vi "Calc Currente Exposure Time.vi"(8 "error in (no error)":errorcluster, 11 "CCDCamera in":refnum<class "Simulated_CCD_Camera.lvclass">) -> (0 "error out":errorcluster, 3 "CCDCamera out":refnum<class "Simulated_CCD_Camera.lvclass">)   [LabVIEW 2018, in "Simulated_CCD_Camera.lvclass"]
doc: "Calculate the exposure time of the current acquisition\n\nThis calculation is based on the timestamp get after the star of the acquisition"
uses:
  Simulated_CCD_Camera.lvclass
  Simulated_CCD_Camera.lvclass/Simulated_CCD_Camera.ctl
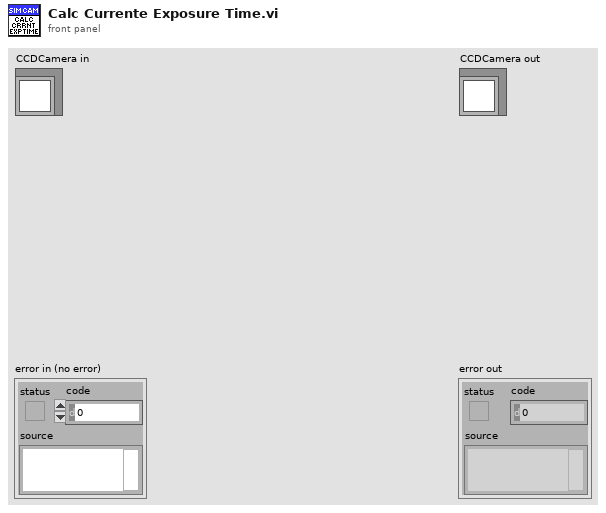
[diagram p1: front panel]
types:
  T1 = cluster{"CYCLES_DONE":u16, "LAST_IMAGE_NAME":string, "DISK_SPACE":u16, "FRAMES_DONE":u16, "CCD_STATUS":string, "CURRENT_TEMPERATURE":i16, "TEMPERATURE_STATUS":string, "FRAME_EXPOSURE_TIME":sgl, "ERROR":bool, "SERIAL_NUMBER":u16, "ACQUIRING":bool, "IMAGE_INDEX":u32, "SEQS_DONE":u16}
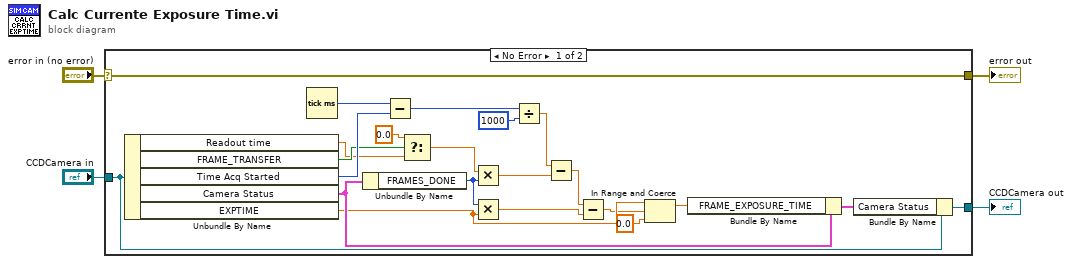
[diagram p0: block diagram]
diagram:
  n1 = case shown="No Error" "error in (no error)" {
    selector: "error in (no error)" -> [w6 w28]
    tunnel: [w6 w28] -> w3
    tunnel: [w26 w27] -> w1
    tunnel: "CCDCamera in" -> [w13 w27]
    frame No Error {
      n2 = Unbundle By Name(w13) -> ("Readout time"=w5:dbl, "FRAME_TRANSFER"=w14:bool, "Time Acq Started"=w24:u32, "Camera Status"=w21:T1, "EXPTIME"=w19:dbl)
      n3 = Tick Count (ms)() -> (millisecond timer value=w25:u32)
      n4 = Unbundle By Name(w21) -> ("FRAMES_DONE"=w7:u16)
      n5 = Subtract(x=w25, y=w24) -> (x-y=w23:u32)
      n6 = Select(t=sgl 0.0, s=w14, f=w5) -> (s? t:f=w9:dbl)
      n7 = Multiply(x=w9, y=w7) -> (x*y=w8:dbl)
      n8 = Multiply(x=w7, y=w19) -> (x*y=w17:dbl)
      n9 = Divide(x=w23, y=1000) -> (x/y=w11:dbl)
      n10 = Subtract(x=w11, y=w8) -> (x-y=w10:dbl)
      n11 = Subtract(x=w10, y=w17) -> (x-y=w16:dbl)
      n12 = In Range and Coerce(upper limit=w19, x=w16, lower limit=sgl 0.0) -> (coerced(x)=w12:dbl)  [unwired: 1 out]
      n13 = Bundle By Name(cluster=w21, "FRAME_EXPOSURE_TIME"=w12) -> (w20:T1)
      n14 = Bundle By Name(cluster=w13, "Camera Status"=w20) -> (w26:refnum<class "Simulated_CCD_Camera.lvclass">)
    }
    frame Error {
    }
  }
  "error out" <- w3
  "CCDCamera out" <- w1
